vi "FlatToRichni_measurementlink_measurement_v1_UserInterfaceDetails.vi"(5 "OutputClusterType":T1, 11 "InputCluster":T2) -> (3 "OutputCluster":T1)   [LabVIEW 2021, in "ni.measurementlink.measurement.v1.api.lvlib"]
uses:
  ni.measurementlink.measurement.v1.api.lvlib
  ni_measurementlink_measurement_v1_UserInterfaceDetails_Flat.ctl
  ni_measurementlink_measurement_v1_UserInterfaceDetails.ctl
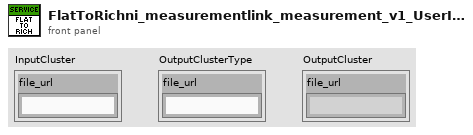
[diagram p1: front panel]
types:
  T1 = typedef "ni.measurementlink.measurement.v1.api.lvlib/ni_measurementlink_measurement_v1_UserInterfaceDetails.ctl" = cluster{"file_url":string}
  T2 = typedef "ni.measurementlink.measurement.v1.api.lvlib/ni_measurementlink_measurement_v1_UserInterfaceDetails_Flat.ctl" = cluster{"file_url":string}
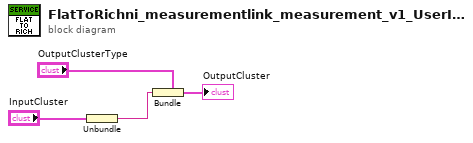
[diagram p0: block diagram]
diagram:
  n1 = Unbundle "Unbundle"("InputCluster") -> ("file_url"=w1:string)
  n2 = Bundle "Bundle"(cluster="OutputClusterType", "file_url"=w1) -> (→"OutputCluster":T1)
